vi "Analog_Delay.vi"(8 "Time":dbl=-1.0, 9 "Delay Time":dbl=1.0, 11 "Input":dbl) -> (1 "IsPresent":bool, 3 "Output":dbl)   [LabVIEW 2019, in "Trajectory_Library.lvlib"]
doc: "This VI implements an analog \"time delay\". The output is the input delayed by \"Delay\" seconds. If the \"Delay\" time does not exactly match the sample period,, the value is calculated by interpolating the nearest buffer samples.\n\nInputs:\n - Input -- Double input value\n - Delay Time -- Time (seconds) to delay the otuput value. If time delay is increaed, then the buffer is re-created. FALSE will be returned until the buffer has sufficient data to return a delayed value.\n - Time -- Continously counting system time, Seconds. If not wired the FPGA time will be used.\n\nOutputs:\n - Output -- Double output value with delay applied\n - IsPresent -- Set to TRUE if the buffer has enough data to return a delayed value."
uses:
  TimeInterpBoolean_CleanUp.vi
  <vilib>/gmath/interp.llb/Search Ordered Table.vi
  Trajectory_Library.lvlib
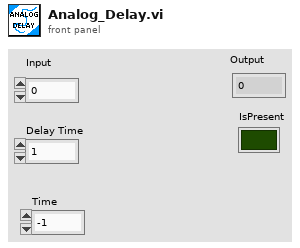
[diagram p1: front panel]
types:
  T1 = typedef "Trajectory_Library.lvlib/TIME_INTERPOLATABLE_DOUBLE.ctl" = cluster{"TimeStamps":dbl[], "DoubleValue":dbl[], "Min_TimeStamp":dbl, "Max_TimeStamp":dbl, "ItemCount":i32, "MaxBufferTime":dbl}
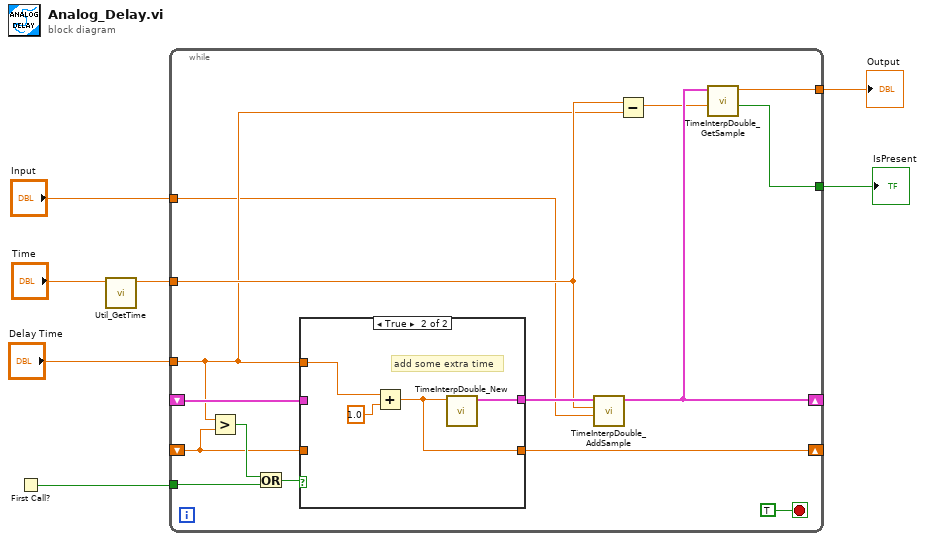
[diagram p0: block diagram]
diagram:
  n1 = First Call?() -> (First Call?: T/F=w6:bool)
  n2 = call "Util_GetTime.vi"("Pass_Through_Time"="Time") -> ("FPGA_Time_Seconds"=w4:dbl)  [unwired: 9 in, 1 out]
  n3 = while {
    tunnel: "Delay Time" -> [w11]
    tunnel: w6 -> [w12]
    shift-right: [w20] -> _
    shift-left: _ -> [w15]
    tunnel: w4 -> [w19]
    tunnel: "Input" -> [w8]
    tunnel: [w17] -> w2
    tunnel: [w16] -> w1
    shift-right: [w14] -> _
    shift-left: _ -> [w9]
    stop <- TRUE stop-if-true
    n4 = Greater?(x=w11, y=w9) -> (0:w10:bool)
    n5 = Or(x=w10, y=w12) -> (x .or. y?=w13:bool)
    n6 = case shown="True" w13 {
      tunnel: w11 -> [_ w26]
      tunnel: [w24 w27] -> w21
      tunnel: w15 -> [w24 _]
      tunnel: [w23 w25] -> w14
      tunnel: w9 -> [w23 _]
      frame False {
      }
      frame True {
        # "add some extra time"
        n7 = Add(x=w26, y=1.0) -> (x+y=w25:dbl)
        n8 = call "TimeInterpDouble_New.vi"("MaxTime"=w25) -> ("TimeInterpDouble"=w27:T1)  [unwired: 10 in]
      }
    }
    n9 = call "TimeInterpDouble_AddSample.vi"("Value"=w8, "TimeStamp"=w19, "in TimeInterpDouble"=w21) -> ("out TimeInterpDouble"=w20:T1)  [unwired: 7 in, 1 out]
    n10 = Subtract(x=w19, y=w11) -> (x-y=w18:dbl)
    n11 = call "TimeInterpDouble_GetSample.vi"("TimeStamp"=w18, "TimeInterpDouble"=w20) -> ("IsPresent"=w16:bool, "OutputDouble"=w17:dbl)  [unwired: 8 in]
  }
  "Output" <- w2
  "IsPresent" <- w1
